vi "Feeding.vi"(8 "error In":errorcluster) -> (0 "error out":errorcluster)   [LabVIEW 2017]
uses:
  Controls/LOADING_DISPLAY.ctl
  <vilib>/Utility/error.llb/DialogType.ctl
  Controls/Feed_Cyc_Data.ctl
  Controls/QUEUE_STATES.ctl
  Controls/Feed_St.ctl
  <vilib>/Utility/file.llb/Read Delimited Spreadsheet (string).vi
  <vilib>/Instr/_visa.llb/VISA Configure Serial Port (Instr).vi
panel:
  out "ALL DOOR CLOSED":bool
  out "all rows":string[][](array[string])
  out "element":u16
  out "Boolean array":bool[](array[boolean])
  out "output cluster 2":cluster{"RECIPE INDEX":i32, "COMBI BIN":i32}
  in  "Close _Door":bool
  out "raw scan code":string
  in  "BYPASS SCN":bool
  in  "String":string
  out "Scanner Comm":bool
  out "Stop scanner":bool
  out "CYCLE STATUS":string
  out "CURRENT PLAN":T1
  out "SCAN CODE:":string
  out "Selected Plan structure":string[][](table)
  out "Plan Selected:":string
  out "USER:-":string
  in  "Stop":bool
  out "DATE/TIME":string
  out "Screen Name":string
  # "DOOR NUMBER"
  # "SCANNED CODE"
  # "FEEDER STATUS"
  # "DOOR NUMBER"
  # "SCANNED CODE"
  # "FEEDER STATUS"
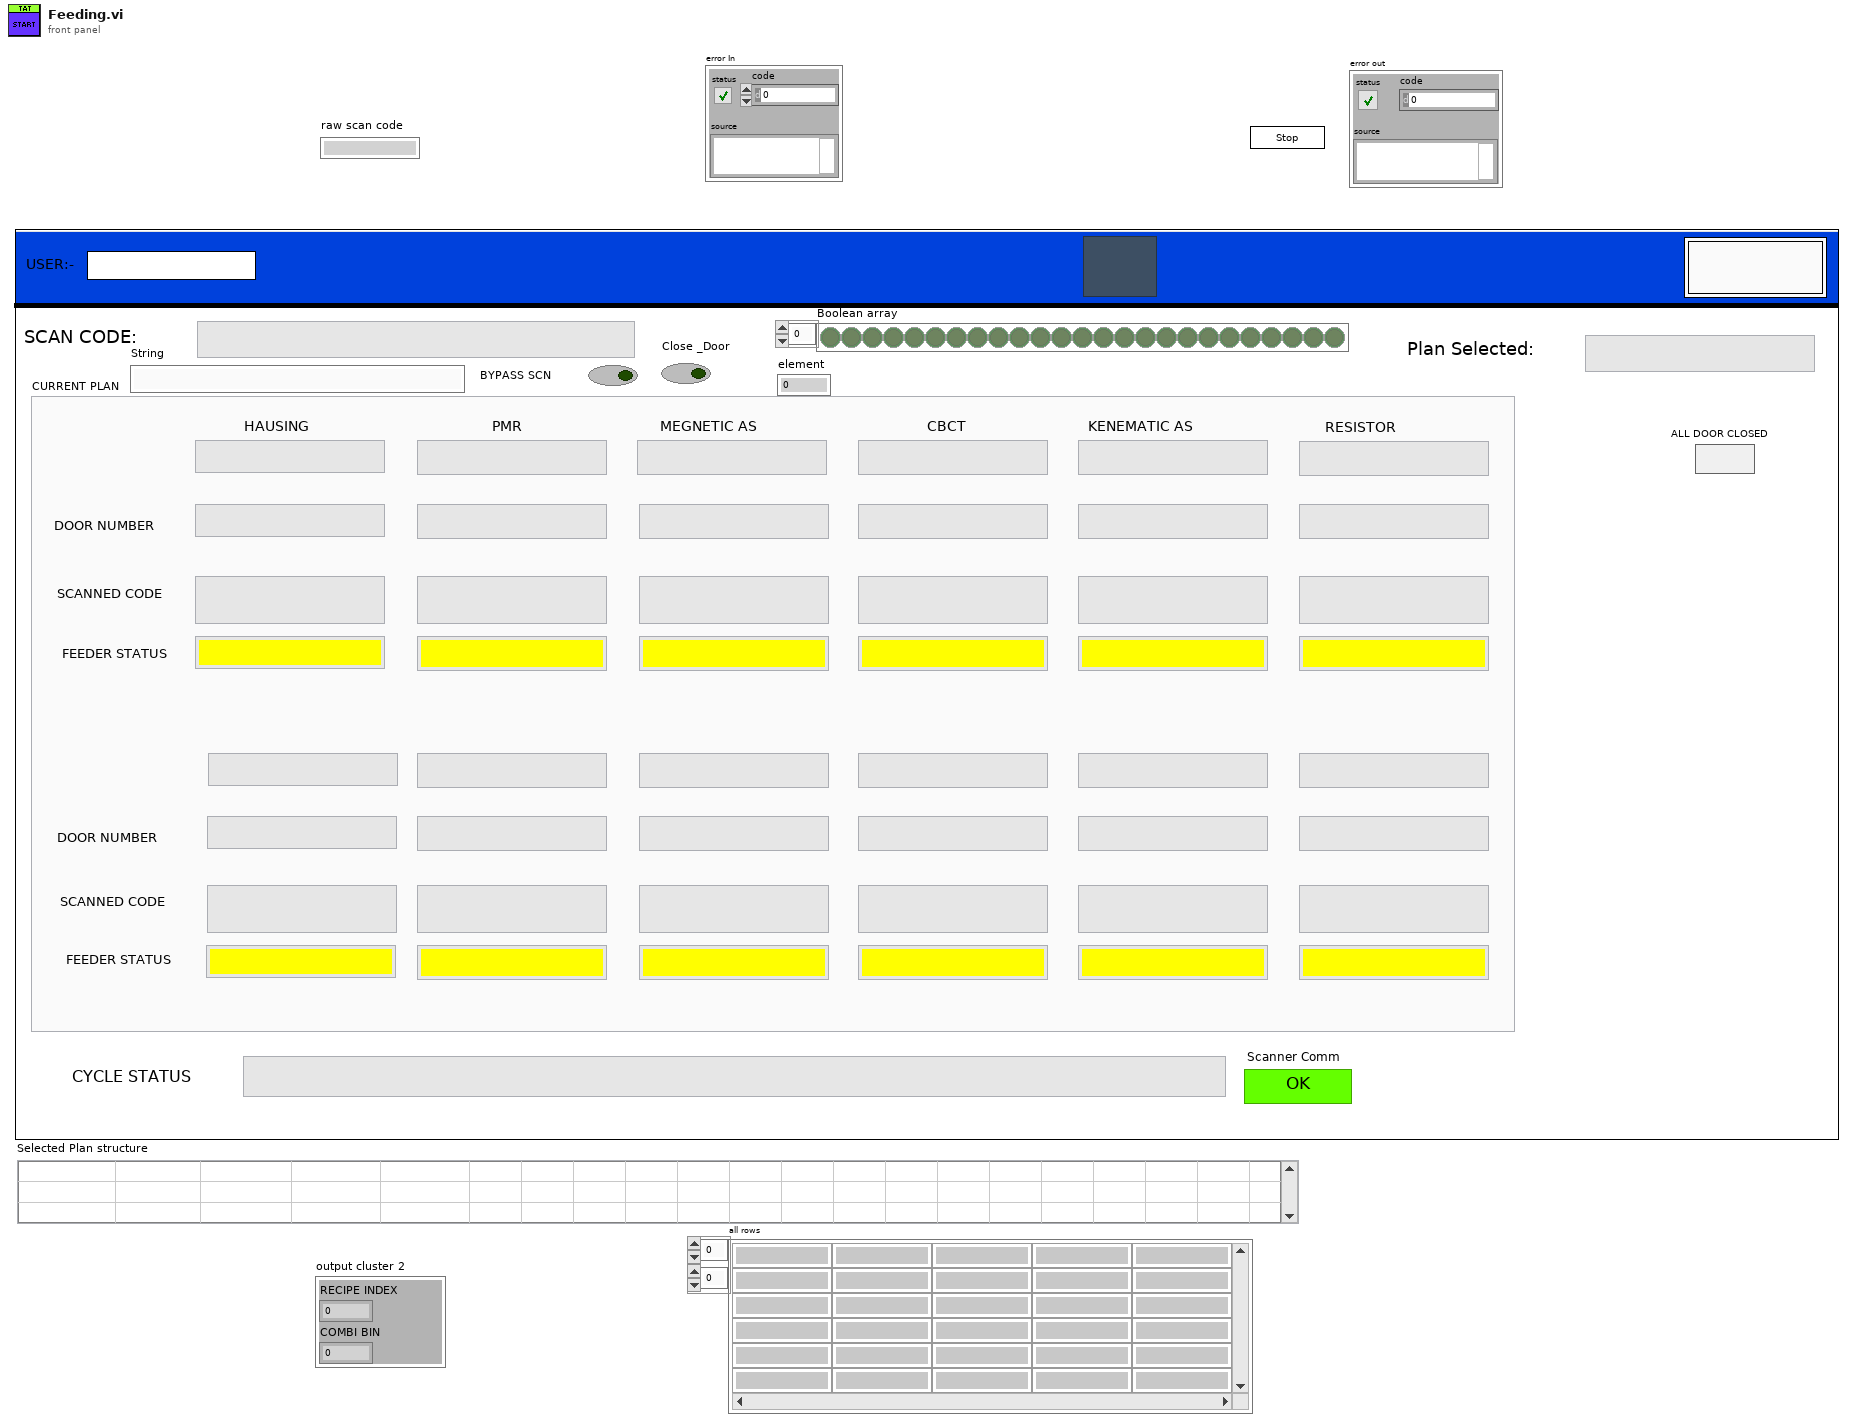
[diagram p1: front panel]
types:
  T1 = typedef "LOADING_DISPLAY.ctl" = cluster{"HAUSING":string, "PMR":string, "MEGNETIC AS":string, "CBCT":string, "KENEMATIC AS":string, "RESISTOR":string, "HAUSING DOOR":string, "PMR DOOR":string, "MAGNETIC AS DOOR":string, "CBCT DOOR":string, "KINEMATIC AS DOOR":string, "RESISTOR DOOR":string, "HAUSING SCAN QR":string, "PMR SCAN QR":string, "MAGNETIC SCAN QR":string, "CBCT SCAN QR":string, "KINEMATIC SCAN QR":string, "RESISTOR SCAN QR":string, "HAUSING FEED STATUS":string, "PMR FEED STATUS":string, "MAGNETIC AS FEEED STATUS":string, "CBCT FEED STATUS":string, "KINEMATIC AS FEED STATUS":string, "RESISTOR 1 FEED STATUS":string, "HAUSING 2":string, "PMR 2":string, "MEGNETIC AS 2":string, "CBCT 2":string, "KENEMATIC AS 2":string, "RESISTOR 2":string, "HAUSING DOOR 4":string, "PMR DOOR 4":string, "MAGNETIC AS DOOR 4":string, "CBCT DOOR 4":string, "KINEMATIC AS DOOR 4":string, "RESISTOR 1 DOOR 4":string, "HAUSING 2 SCAN QR":string, "PMR 2 SCAN QR":string, "MAGNETIC 2 SCAN QR":string, "CBCT 2 SCAN QR":string, "KINEMATIC 2 SCAN QR":string, "RESISTOR 2 SCAN QR":string, "HAUSING FEED STATUS 2":string, "PMR FEED STATUS 2":string, "MAGNETIC AS FEEED STATUS 2":string, "CBCT FEED STATUS 2":string, "KINEMATIC AS FEED STATUS 2":string, "RESISTOR 1 FEED STATUS 2":string}
  T2 = typedef "Feed_Cyc_Data.ctl" = cluster{"Cycle_Plan":path, "Plan_Data":string[][], "Scanned_Data":string[], "Scanned Chld Part":cluster{"Selected Door No":string, "child part code":string, "chld prt Row":i32, "Chld Prt Index":i32, "Scanned Data":string}, "feed Status Indi":refnum<vi>[], "Recipe Selected":cluster{"SELTED RECP & COMBI BIN":cluster{i32, i32}, "SELECTED RECIPE":string}, "CYCLE STATUS":string}
  T3 = typedef "DialogType.ctl" = u16
  T4 = enum32{"invalid app kind", "Development System", "Run Time System", "Student Edition", "Embedded LabVIEW", "Evaluation", "Custom"}
  T5 = typedef "QUEUE_STATES.ctl" = enum16{"CREATE Q", "EN Q", "DE Q", "CLOSE Q"}
  T6 = cluster{"Printer IP":string, "PLC IP Address":string, "Scanner Com":refnum<visa-resource-name>}
  T7 = typedef "Feed_St.ctl" = enum16{"Int 2", "Cluster_update", "Read_Plan", "QR_Scanned", "Int", "SaveReport ", "Error_Handler", "Wait", "Close_Door", "Stop"}
  T8 = cluster{"Selected Door No":string, "child part code":string, "chld prt Row":i32, "Chld Prt Index":i32, "Scanned Data":string}
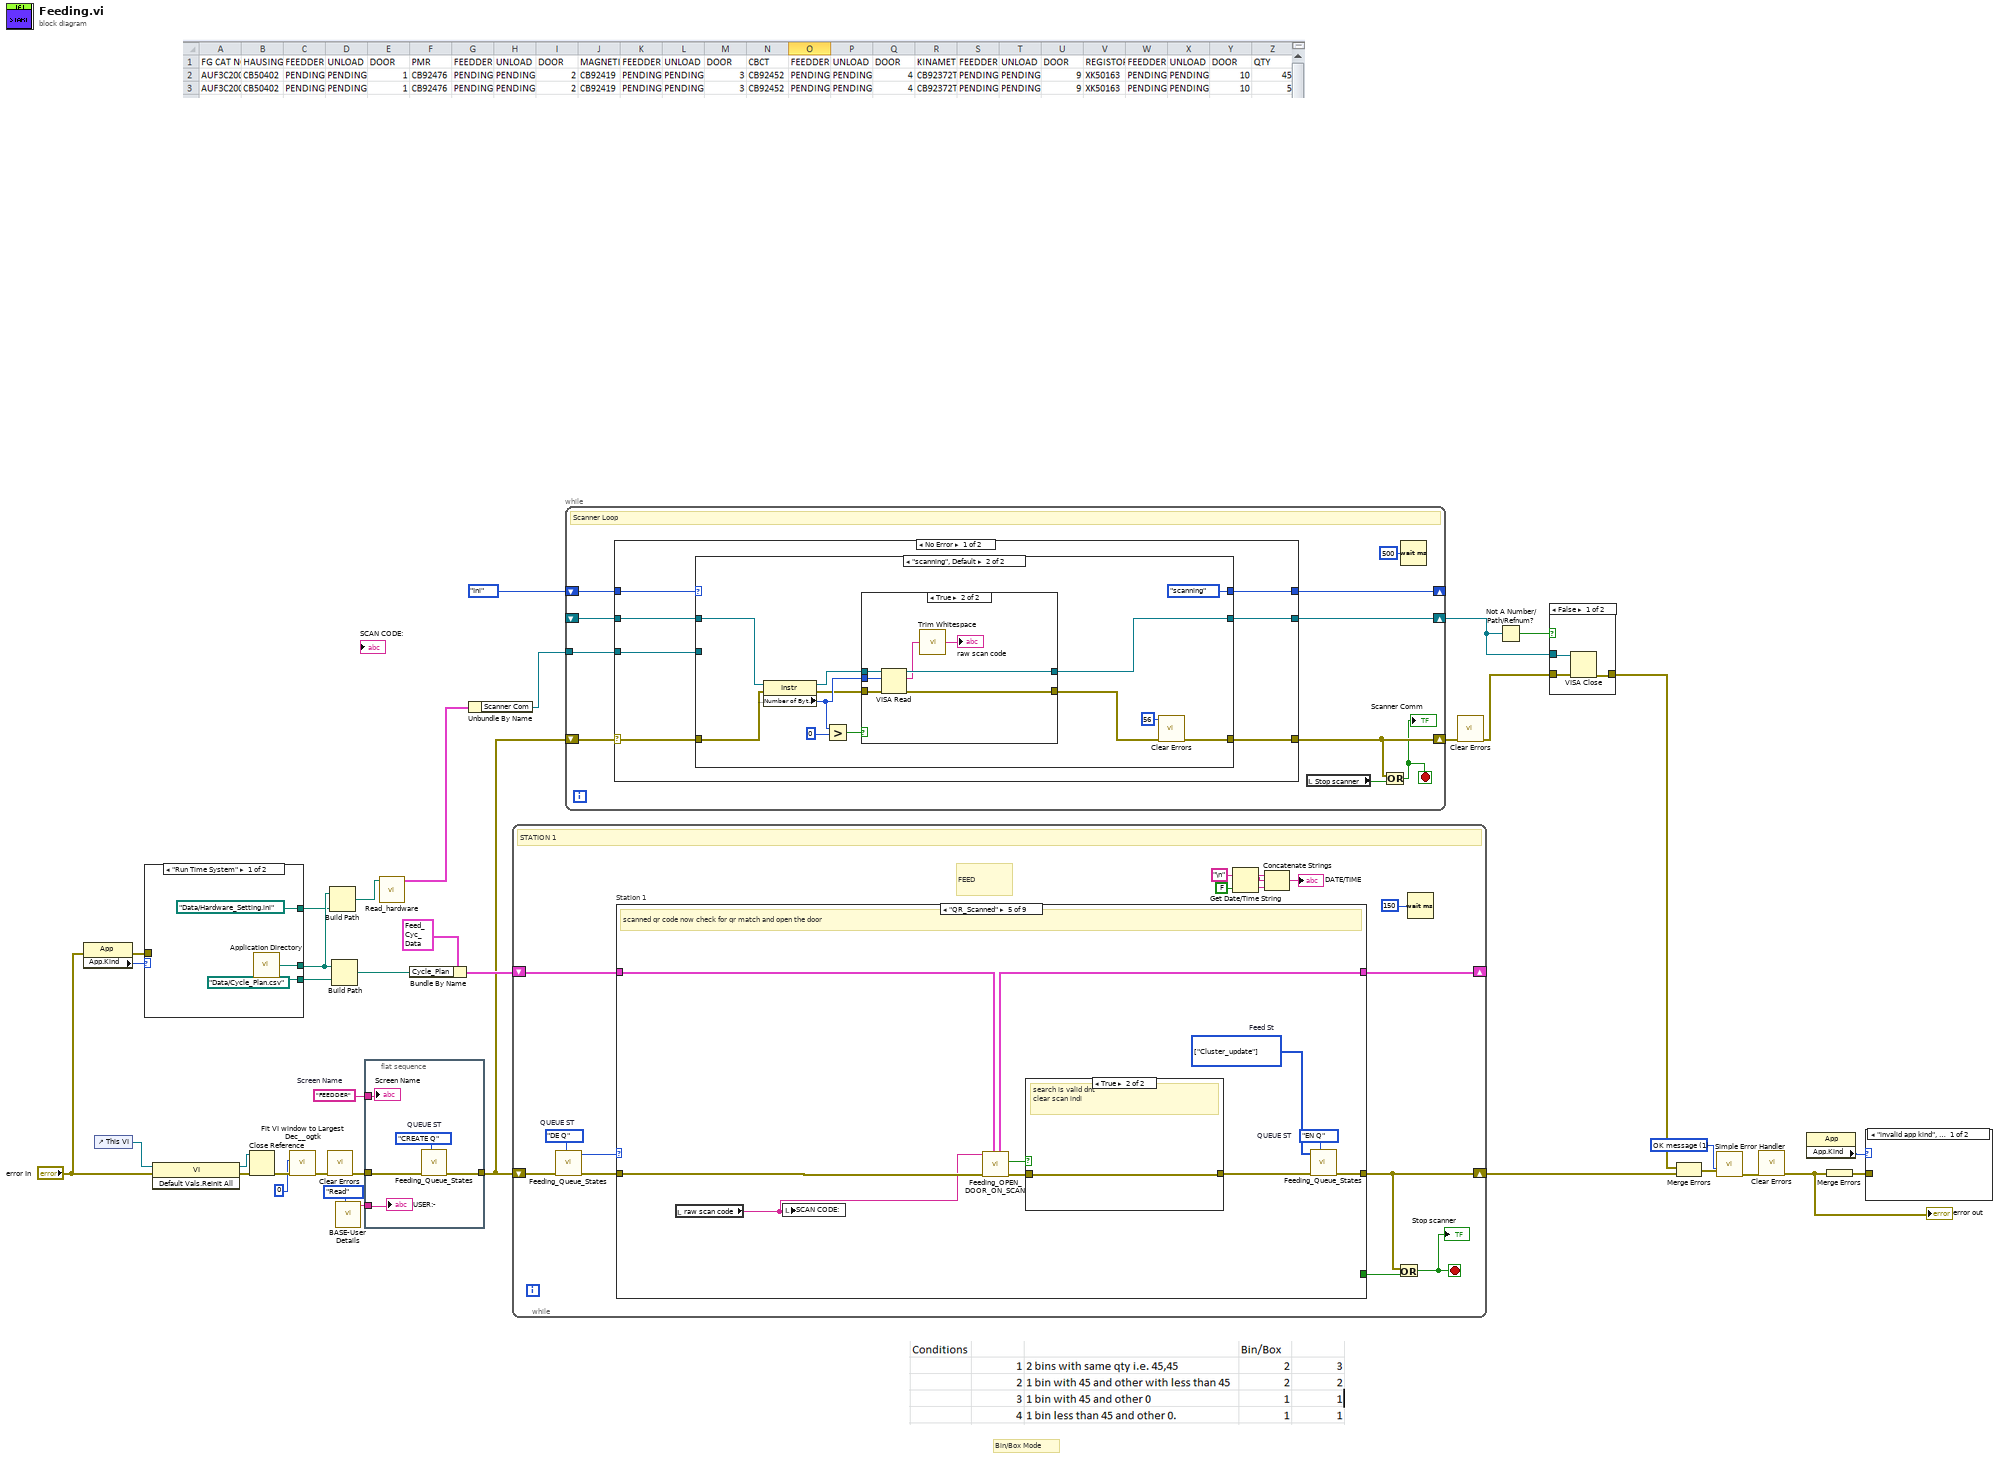
[diagram p0: block diagram]
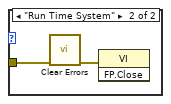
[diagram p2: hidden frame]
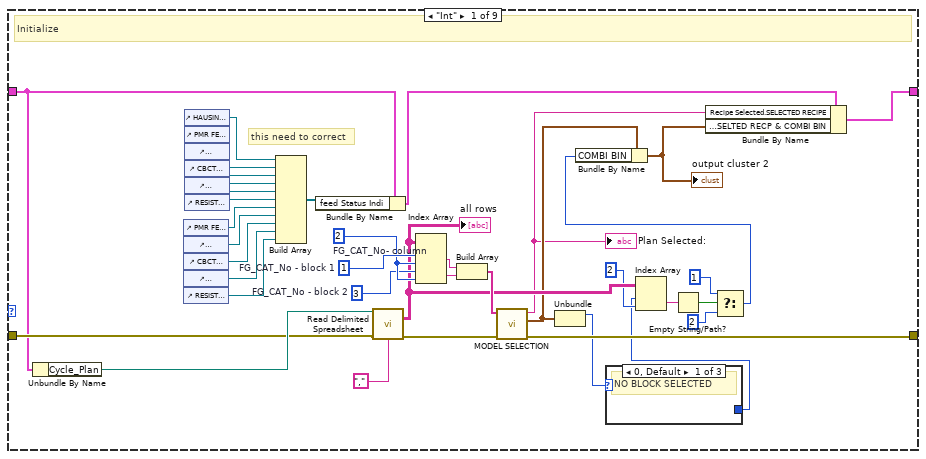
[diagram p3: hidden frame]
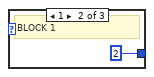
[diagram p4: hidden frame]
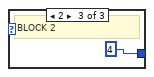
[diagram p5: hidden frame]
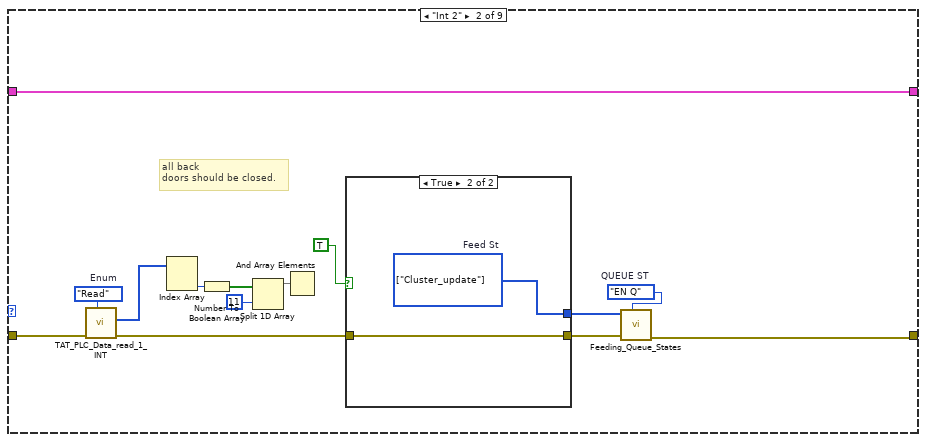
[diagram p6: hidden frame]
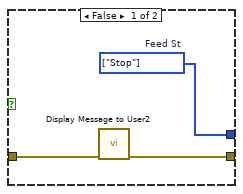
[diagram p7: hidden frame]
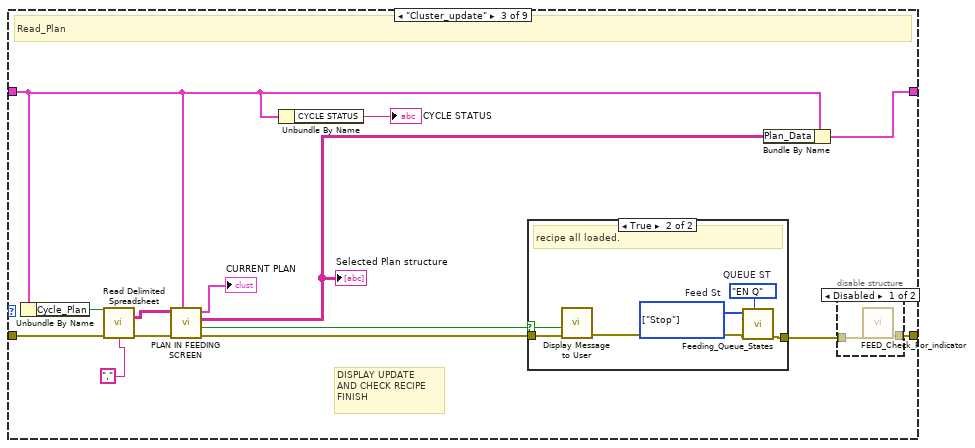
[diagram p8: hidden frame]
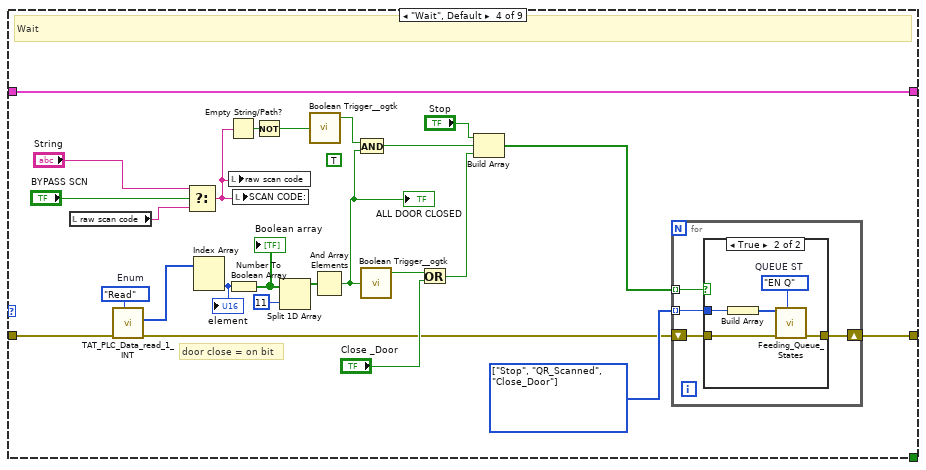
[diagram p11: hidden frame]
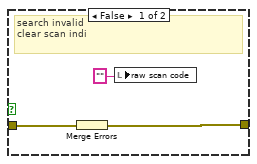
[diagram p13: hidden frame]
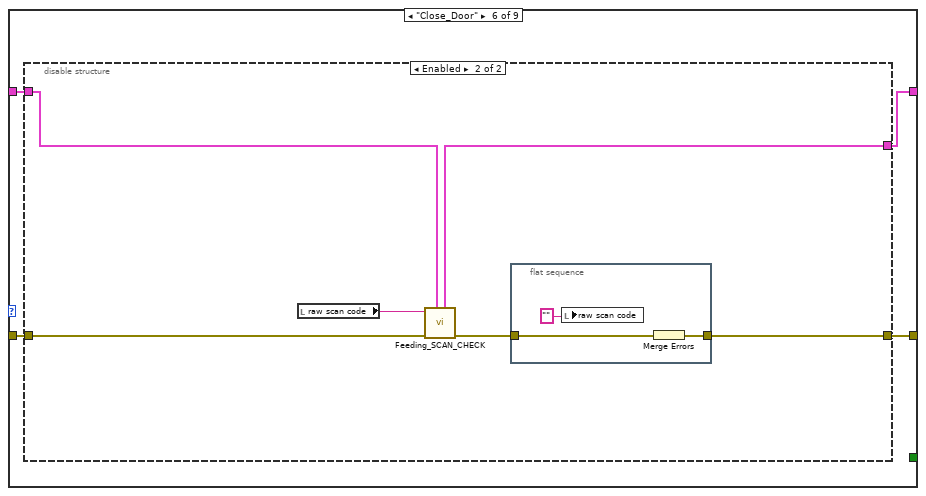
[diagram p14: hidden frame]
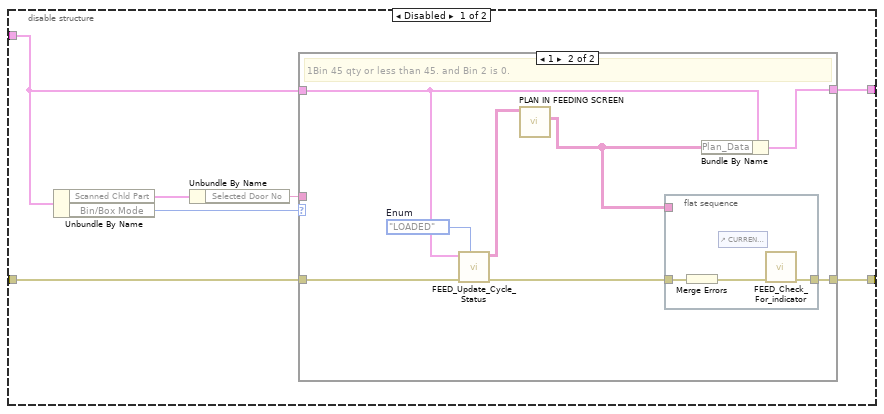
[diagram p15: hidden frame]
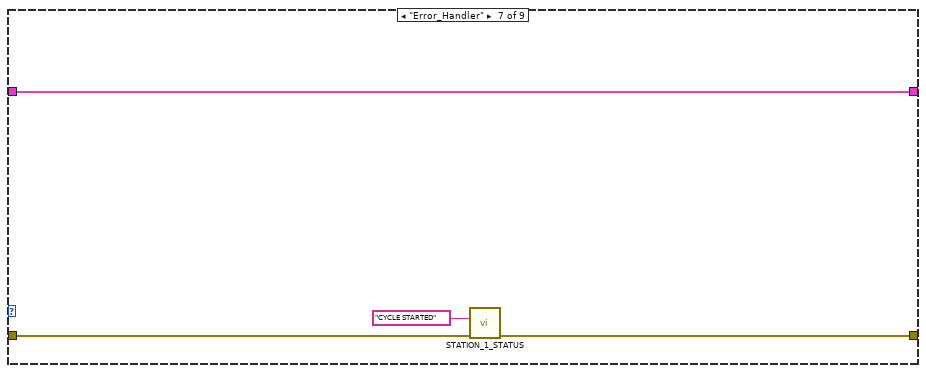
[diagram p17: hidden frame]
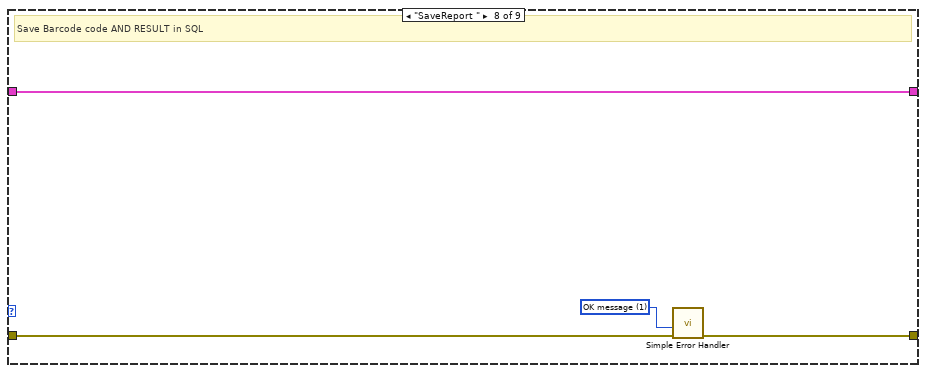
[diagram p18: hidden frame]
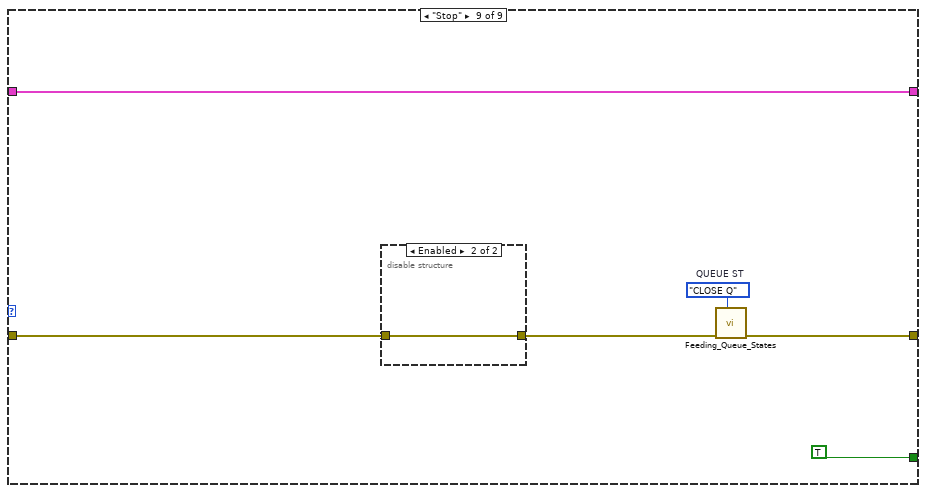
[diagram p19: hidden frame]
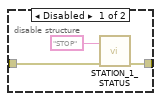
[diagram p20: hidden frame]
diagram:
  w17 = "FEEDDER"  # Screen Name
  w29 = T3 1 items=["no dialog", "OK message", "continue or stop message", "OK message + warnings", "continue/stop + warnings"] ("type of dialog (OK msg:1)")
  # "Bin/Box Mode"
  n1 = property class="App"(error in="error In") -> (error out=w25:errorcluster, "App.Kind"=w27:T4)  [unwired: 1 in, 1 out]
  n2 = control-ref of="This VI"() -> (w36:refnum<vi>)
  n3 = case shown="\"Run Time System\"" w27 {
    tunnel: [path "Data/Cycle_Plan.csv" ("path") path "../Data/Cycle_Plan.csv" ("path")] -> w26
    tunnel: [w37 w41] -> w6
    tunnel: w25 -> [_ _]
    tunnel: [path "Data/Hardware_Setting.ini" ("path") path "../Data/Hardware_Setting.ini" ("path")] -> w5
    frame "Run Time System" {
      n4 = call <vilib>:"Application Directory.vi"() -> ("Application Directory"=w37:path)
    }
    frame Default {
      n5 = Current VI's Path() -> (path=w42:path)
      n6 = Strip Path(path=w42) -> (stripped path=w41:path)  [unwired: 1 out]
    }
  }
  n7 = invoke class="VI" method="Default Vals.Reinit All"(reference=w36, error in="error In") -> (reference out=w34:refnum<vi>, error out=w35:errorcluster)  [unwired: 1 in, 1 out]
  n8 = Close Reference(reference=w34, error in (no error)=w35) -> (error out=w33:errorcluster)
  n9 = call <userlib>:"Fit VI window to Largest Dec__ogtk.vi"("error in (no error)"=w33, "border spacing (2 px)"=0) -> ("error out"=w23:errorcluster)  [unwired: 4 in, 1 out]
  n10 = call <vilib>:"Clear Errors.vi"("error in (no error)"=w23) -> ("error out"=w10:errorcluster)  [unwired: 5 in, 1 out]
  n11 = Build Path(base path=w6, name or relative path=w5) -> (appended path=w4:path)
  n12 = Build Path(base path=w6, name or relative path=w26) -> (appended path=w19:path)
  n13 = call "BASE-User Details.vi"("Enum"=enum16{"Read", "Write"}."Read") -> ("User Name Out"=w30:string)  [unwired: 9 in, 1 out]
  n14 = flat-sequence {
    tunnel: [w45] -> w11
    tunnel: w10 -> [w46]
    tunnel: w30 -> [w48]
    tunnel: w17 -> [w47]
    frame #0 {
      w44 = QUEUE_STATES."CREATE Q"  # QUEUE ST
      n15 = call "Feeding_Queue_States.vi"("QUEUE ST"=w44, "error in"=w46) -> ("error OUT"=w45:errorcluster)  [unwired: 8 in, 1 out]
      "USER:-" <- w48
      "Screen Name" <- w47
    }
  }
  n16 = call "Read_hardware.vi"("configuration file path"=w4) -> ("data"=w8:T6)  [unwired: 10 in]
  n17 = Bundle By Name(cluster=T2 {"Cycle_Plan"=path "", "Plan_Data"=[], "Scanned_Data"=[], "Scanned Chld Part"={"Selected Door No"="", "child part code"="", "chld prt Row"=0, "Chld Prt Index"=0, "Scanned Data"=""}, "feed Status Indi"=[], "Recipe Selected"={"SELTED RECP & COMBI BIN"={0, 0}, "SELECTED RECIPE"=""}, "CYCLE STATUS"=""}, "Cycle_Plan"=w19) -> (w18:T2)
  n18 = Unbundle By Name(w8) -> ("Scanner Com"=w7:refnum<visa-resource-name>)
  n19 = while {
    shift-right: [w55] -> _
    shift-left: w18 -> [w56]
    shift-right: [w53] -> w9
    shift-left: w11 -> [w52]
    stop <- w54 stop-if-true
    w50 = QUEUE_STATES."DE Q"  # QUEUE ST
    # "FEED"
    # "STATION 1"
    n20 = call "Feeding_Queue_States.vi"("QUEUE ST"=w50, "error in"=w52) -> ("error OUT"=w51:errorcluster, "Feed ST"=w49:T7)  [unwired: 8 in]
    n21 = case "Station 1" shown="\"QR_Scanned\"" w49 {
      tunnel: [_ _ _ _ _ _ _ _ TRUE] -> w57
      tunnel: [w67 w106 w130 w168 w183 w198 w230 w235 w237] -> w53
      tunnel: w51 -> [w86 w110 w135 w157 w191 w199 w231 w234 w241]
      tunnel: w56 -> [w77 w117 w124 w171 w188 w197 w229 w233 w240]
      tunnel: [w78 w117 w129 w171 w187 w196 w229 w233 w240] -> w55
      frame "Int" {
        w82 = 3  # FG_CAT_No - block 2
        w84 = 1  # FG_CAT_No - block 1
        w83 = 2  # FG_CAT_No- column
        # "this need to correct"
        # "Initialize"
        n22 = Unbundle By Name(w77) -> ("Cycle_Plan"=w89:path)
        n23 = control-ref of="PMR FEED STATUS 2"() -> (w97:refnum<vi>)
        n24 = control-ref of="MAGNETIC AS FEEED STATUS 2"() -> (w98:refnum<vi>)
        n25 = control-ref of="CBCT FEED STATUS 2"() -> (w99:refnum<vi>)
        n26 = control-ref of="KINEMATIC AS FEED STATUS 2"() -> (w100:refnum<vi>)
        n27 = control-ref of="RESISTOR 1 FEED STATUS 2"() -> (w101:refnum<vi>)
        n28 = control-ref of="HAUSING FEED STATUS"() -> (w91:refnum<vi>)
        n29 = control-ref of="PMR FEED STATUS"() -> (w92:refnum<vi>)
        n30 = control-ref of="MAGNETIC AS FEEED STATUS"() -> (w93:refnum<vi>)
        n31 = control-ref of="CBCT FEED STATUS"() -> (w94:refnum<vi>)
        n32 = control-ref of="KINEMATIC AS FEED STATUS"() -> (w95:refnum<vi>)
        n33 = control-ref of="RESISTOR 1 FEED STATUS"() -> (w96:refnum<vi>)
        n34 = Build Array(w91, w92, w93, w94, w95, w96, w97, w98, w99, w100, w101) -> (w90:refnum<vi>[])
        n35 = Bundle By Name(cluster=w77, "feed Status Indi"=w90) -> (w79:T2)
        n36 = call-poly <vilib>:"Read Delimited Spreadsheet.vi"("file path (dialog if empty)"=w89, "error in (no error)"=w86, "delimiter (\\t)"=",") -> ("all rows"=w76:string[][], "error out"=w85:errorcluster)  [unwired: 7 in, 4 out]
        "all rows" <- w76
        n37 = Index Array(array=w76, index (row) #1=w84, index (col) #1=w83, index (row) #2=w82, index (col) #2=w83) -> (element #1=w81:string, element #2=w80:string)
        n38 = Build Array(w81, w80) -> (w88:string[])
        n39 = call "MODEL SELECTION.vi"("error in (no error)"=w85, "Plan List"=w88) -> ("error out 2"=w67:errorcluster, "SELECTED RECIPE\nand COMBI OF BIN- INDEX"=w70:cluster{"RECIPE INDEX":i32, "COMBI BIN":i32}, "Plan Selected"=w68:string)  [unwired: 7 in]
        "Plan Selected:" <- w68
        n40 = Unbundle(w70) -> ("RECIPE INDEX"=w66:i32)  [unwired: 1 out]
        n41 = case shown="0, Default" w66 {
          tunnel: [_ 2 4] -> w64
          frame 0, Default {
            # "NO BLOCK SELECTED"
          }
          frame 1 {
            # "BLOCK 1"
          }
          frame 2 {
            # "BLOCK 2"
          }
        }
        n42 = Index Array(array=w76, index (row)=w64, index (col)=2) -> (element=w74:string)
        n43 = Empty String/Path?(string/path=w74) -> (empty?=w73:bool)
        n44 = Select(t=1, s=w73, f=2) -> (s? t:f=w65:i32)
        n45 = Bundle By Name(cluster=w70, "COMBI BIN"=w65) -> (w69:cluster{"RECIPE INDEX":i32, "COMBI BIN":i32})
        "output cluster 2" <- w69
        n46 = Bundle By Name(cluster=w79, "Recipe Selected.SELECTED RECIPE"=w68, "Recipe Selected.SELTED RECP & COMBI BIN"=w69) -> (w78:T2)
      }
      frame "Int 2" {
        w108 = QUEUE_STATES."EN Q"  # QUEUE ST
        w116 = enum16{"Read", "Write"}."Read"  # Enum
        # "all back\ndoors should be closed."
        n47 = call "TAT_PLC_Data_read_1_INT.vi"("Enum"=w116, "error in (no error)"=w110) -> ("error out"=w109:errorcluster, "Array 2"=w115:u16[])  [unwired: 8 in]
        n48 = Index Array(array=w115) -> (element #2=w114:u16)  [unwired: 2 in, 1 out]
        n49 = Number To Boolean Array(number=w114) -> (Boolean array=w113:bool[])
        n50 = Split 1D Array(array=w113, index=11) -> (first subarray=w111:bool[])  [unwired: 1 out]
        n51 = And Array Elements(Boolean array=w111) -> ()  [unwired: 1 out]
        n52 = case shown="True" TRUE {
          tunnel: w109 -> [w119 w121]
          tunnel: [w118 w121] -> w105
          tunnel: [w120 w122] -> w107
          frame False {
            w120 = T7[] [enum."Stop"] items=["Int 2", "Cluster_update", "Read_Plan", "QR_Scanned", "Int", "SaveReport ", "Error_Handler", "Wait", "Close_Door", "Stop"]  # Feed St
            n53 = call "Display Message to User2"("error in (no error)"=w119) -> ("error out"=w118:errorcluster)  [unwired: 9 in, 1 out]
          }
          frame True {
            w122 = T7[] [enum."Cluster_update"] items=["Int 2", "Cluster_update", "Read_Plan", "QR_Scanned", "Int", "SaveReport ", "Error_Handler", "Wait", "Close_Door", "Stop"]  # Feed St
          }
        }
        n54 = call "Feeding_Queue_States.vi"("QUEUE ST"=w108, "error in"=w105, "Feed St"=w107) -> ("error OUT"=w106:errorcluster)  [unwired: 7 in, 1 out]
      }
      frame "Cluster_update" {
        # "DISPLAY UPDATE\nAND CHECK RECIPE\nFINISH"
        # "Read_Plan"
        n55 = Unbundle By Name(w124) -> ("Cycle_Plan"=w134:path)
        n56 = call-poly <vilib>:"Read Delimited Spreadsheet.vi"("file path (dialog if empty)"=w134, "error in (no error)"=w135, "delimiter (\\t)"=",") -> ("all rows"=w132:string[][], "error out"=w127:errorcluster)  [unwired: 7 in, 4 out]
        n57 = call "PLAN IN FEEDING SCREEN.vi"("LOOP DATA IN"=w124, "error IN"=w127, "PLAN In"=w132) -> ("error out"=w128:errorcluster, "NO EMPTY CMPLT?"=w125:bool, "PLAN Out"=w133:string[][], "CURRENT PLAN"=→"CURRENT PLAN":T1)  [unwired: 4 in]
        "Selected Plan structure" <- w133
        n58 = Unbundle By Name(w124) -> ("CYCLE STATUS"=→"CYCLE STATUS":string)
        n59 = case shown="True" w125 {
          selector: w125 -> [_ w141]
          tunnel: w128 -> [w140 w143]
          tunnel: [w140 w145] -> w131
          frame False {
          }
          frame True {
            w144 = T7[] [enum."Stop"] items=["Int 2", "Cluster_update", "Read_Plan", "QR_Scanned", "Int", "SaveReport ", "Error_Handler", "Wait", "Close_Door", "Stop"]  # Feed St
            w146 = QUEUE_STATES."EN Q"  # QUEUE ST
            # "recipe all loaded."
            n60 = call "Display Message to User"("error in (no error)"=w143, "Enable"=w141) -> ("error out"=w142:errorcluster)  [unwired: 8 in, 1 out]
            n61 = call "Feeding_Queue_States.vi"("QUEUE ST"=w146, "error in"=w142, "Feed St"=w144) -> ("error OUT"=w145:errorcluster)  [unwired: 7 in, 1 out]
          }
        }
        n62 = Bundle By Name(cluster=w124, "Plan_Data"=w133) -> (w129:T2)
        n63 = disable-structure shown="Disabled" {
          disable-tunnel: w131 -> [w138 w139]
          disable-tunnel: [w137 w139] -> w130
          frame Disabled {
            n64 = call "FEED_Check_For_indicator.vi"("error in (no error)"=w138) -> ("error out"=w137:errorcluster)  [unwired: 10 in]
          }
          frame Enabled {
          }
        }
      }
      frame "Wait", Default {
        (unwired) TRUE
        w155 = enum16{"Read", "Write"}."Read"  # Enum
        w164 = T7[] [enum."Stop", enum."QR_Scanned", enum."Close_Door"] items=["Int 2", "Cluster_update", "Read_Plan", "QR_Scanned", "Int", "SaveReport ", "Error_Handler", "Wait", "Close_Door", "Stop"] ("Array")
        # "door close = on bit"
        # "Wait"
        n65 = local read "raw scan code"() -> (w163:string)
        n66 = call "TAT_PLC_Data_read_1_INT.vi"("Enum"=w155, "error in (no error)"=w157) -> ("error out"=w156:errorcluster, "Array 2"=w154:u16[])  [unwired: 8 in]
        n67 = Select(t="String", s="BYPASS SCN", f=w163) -> (s? t:f=w160:string)
        n68 = Index Array(array=w154) -> (element #2=w151:u16)  [unwired: 2 in, 1 out]
        "element" <- w151
        n69 = Empty String/Path?(string/path=w160) -> (empty?=w167:bool)
        n70 = local write "raw scan code"(w160) -> ()
        n71 = Number To Boolean Array(number=w151) -> (Boolean array=w150:bool[])
        "Boolean array" <- w150
        n72 = local write "SCAN CODE:"(w160) -> ()
        n73 = Not(x=w167) -> (.not. x?=w159:bool)
        n74 = Split 1D Array(array=w150, index=11) -> (first subarray=w148:bool[])  [unwired: 1 out]
        n75 = call <userlib>:"Boolean Trigger__ogtk.vi"("Boolean Input"=w159) -> ("Rising Edge"=w158:bool)  [unwired: 1 in, 1 out]
        n76 = And Array Elements(Boolean array=w148) -> (logical AND=w147:bool)
        "ALL DOOR CLOSED" <- w147
        n77 = And(x=w158, y=w147) -> (x .and. y?=w153:bool)
        n78 = call <userlib>:"Boolean Trigger__ogtk.vi"("Boolean Input"=w147) -> ("Rising Edge"=w152:bool)  [unwired: 1 in, 1 out]
        n79 = Or(x=w152, y="Close _Door") -> (x .or. y?=w161:bool)
        n80 = Build Array("Stop", w153, w161) -> (w165:bool[])
        n81 = for {
          shift-right: [w174] -> w168
          shift-left: w156 -> [w175]
          tunnel: w165 -> [w173] mode=indexing
          tunnel: w164 -> [w172] mode=indexing
          n82 = case shown="True" w173 {
            tunnel: w175 -> [w176 w180]
            tunnel: [w176 w179] -> w174
            tunnel: w172 -> [_ w178]
            frame False {
            }
            frame True {
              w181 = QUEUE_STATES."EN Q"  # QUEUE ST
              n83 = Build Array(w178) -> (w177:T7[])
              n84 = call "Feeding_Queue_States.vi"("QUEUE ST"=w181, "error in"=w180, "Feed St"=w177) -> ("error OUT"=w179:errorcluster)  [unwired: 7 in, 1 out]
            }
          }
        }
      }
      frame "QR_Scanned" {
        w184 = T7[] [enum."Cluster_update"] items=["Int 2", "Cluster_update", "Read_Plan", "QR_Scanned", "Int", "SaveReport ", "Error_Handler", "Wait", "Close_Door", "Stop"]  # Feed St
        w185 = QUEUE_STATES."EN Q"  # QUEUE ST
        # "scanned qr code now check for qr match and open the door"
        n85 = local read "raw scan code"() -> (w189:string)
        n86 = local write "SCAN CODE:"(w189) -> ()
        n87 = call "Feeding_OPEN_DOOR_ON_SCAN.vi"("CYCLE DATA IN"=w188, "error in (no error)"=w191, "raw scan code"=w189) -> ("error out"=w190:errorcluster, "search valid ?"=w186:bool, "CYCLE DATA OUT"=w187:T2)  [unwired: 6 in]
        n88 = case shown="True" w186 {
          tunnel: w190 -> [w194 w195]
          tunnel: [w193 w195] -> w182
          frame False {
            # "search invalid\nclear scan indi"
            n89 = Merge Errors(w194) -> (w193:errorcluster)
            n90 = local write "raw scan code"("") -> ()
          }
          frame True {
            # "search is valid dnt\nclear scan indi"
          }
        }
        n91 = call "Feeding_Queue_States.vi"("QUEUE ST"=w185, "error in"=w182, "Feed St"=w184) -> ("error OUT"=w183:errorcluster)  [unwired: 7 in, 1 out]
      }
      frame "Close_Door" {
        n92 = disable-structure shown="Enabled" {
          disable-tunnel: w199 -> [w206 w225]
          disable-tunnel: [w205 w220] -> w198
          disable-tunnel: w197 -> [w202 w223]
          disable-tunnel: [w201 w222] -> w196
          frame Disabled {
            n93 = Unbundle By Name(w202) -> ("Scanned Chld Part"=w203:T8, "Bin/Box Mode"=w200:i32)
            n94 = Unbundle By Name(w203) -> ("Selected Door No"=w204:string)
            n95 = case shown="1" w200 {
              tunnel: w206 -> [w207 w215]
              tunnel: [w207 w210] -> w205
              tunnel: w204 -> [_ _]
              tunnel: w202 -> [w208 w212]
              tunnel: [w208 w216] -> w201
              frame 0, Default {
              }
              frame 1 {
                w213 = enum16{"FEED", "LOADED"}."LOADED"  # Enum
                # "1Bin 45 qty or less than 45. and Bin 2 is 0."
                n96 = call "FEED_Update_Cycle_Status.vi"("Enum"=w213, "error in (no error)"=w215, 11:w212) -> ("error out"=w214:errorcluster, "output array"=w211:string[][])  [unwired: 6 in, 1 out]
                n97 = call "PLAN IN FEEDING SCREEN.vi"("PLAN In"=w211) -> ("PLAN Out"=w209:string[][])  [unwired: 6 in, 3 out]
                n98 = flat-sequence {
                  tunnel: w214 -> [w219]
                  tunnel: [w217] -> w210
                  tunnel: w209 -> [_]
                  frame #0 {
                    n99 = Merge Errors(w219) -> (w218:errorcluster)
                    n100 = control-ref of="CURRENT PLAN"() -> ()  [unwired: 1 out]
                    n101 = call "FEED_Check_For_indicator.vi"("error in (no error)"=w218) -> ("error out"=w217:errorcluster)  [unwired: 10 in]
                  }
                }
                n102 = Bundle By Name(cluster=w212, "Plan_Data"=w209) -> (w216:T2)
              }
            }
          }
          frame Enabled {
            n103 = local read "raw scan code"() -> (w221:string)
            n104 = call "Feeding_SCAN_CHECK.vi"("CYCLE DATA IN"=w223, "error in (no error)"=w225, "raw scan code"=w221) -> ("error out"=w224:errorcluster, "CYCLE DATA OUT"=w222:T2)  [unwired: 7 in]
            n105 = flat-sequence {
              tunnel: w224 -> [w228]
              tunnel: [w226] -> w220
              frame #0 {
                n106 = local write "raw scan code"("") -> ()
                n107 = Merge Errors(w228) -> (w226:errorcluster)
              }
            }
          }
        }
      }
      frame "Error_Handler" {
        n108 = call "STATION_1_STATUS.vi"("error in (no error)"=w231, "STATUS"="CYCLE STARTED" ("Cycle Status")) -> ("error out"=w230:errorcluster)  [unwired: 9 in]
      }
      frame "SaveReport " {
        w236 = T3 1 items=["no dialog", "OK message", "continue or stop message", "OK message + warnings", "continue/stop + warnings"] ("type of dialog (OK msg:1)")
        # "Save Barcode code AND RESULT in SQL"
        n109 = call <vilib>:"Simple Error Handler.vi"("type of dialog (OK msg:1)"=w236, "error in (no error)"=w234) -> ("error out"=w235:errorcluster)  [unwired: 3 in, 4 out]
      }
      frame "Stop" {
        w239 = QUEUE_STATES."CLOSE Q"  # QUEUE ST
        n110 = disable-structure shown="Enabled" {
          disable-tunnel: w241 -> [w244 w246]
          disable-tunnel: [w243 w246] -> w238
          frame Disabled {
            n111 = call "STATION_1_STATUS.vi"("error in (no error)"=w244, "STATUS"="STOP" ("Cycle Status")) -> ("error out"=w243:errorcluster)  [unwired: 9 in]
          }
          frame Enabled {
          }
        }
        n112 = call "Feeding_Queue_States.vi"("QUEUE ST"=w239, "error in"=w238) -> ("error OUT"=w237:errorcluster)  [unwired: 8 in, 1 out]
      }
    }
    n113 = Get Date/Time String(want seconds? (F)=FALSE) -> (date string=w61:string, time string=w60:string)  [unwired: 2 in]
    n114 = Concatenate Strings(w61, "\n", w60) -> (→"DATE/TIME":string)
    n115 = Or(x=w53, y=w57) -> (x .or. y?=w54:bool)
    "Stop scanner" <- w54
    n116 = Wait (ms)(milliseconds to wait=u32 150) -> ()  [unwired: 1 out]
  }
  n117 = while {
    shift-right: [w255] -> w15
    shift-left: w11 -> [w256]
    shift-right: [w253] -> _
    shift-left: enum16{"Ini", "scanning", "Close"}."Ini" -> [w254]
    tunnel: w7 -> [w252]
    shift-right: [w251] -> w12
    shift-left: _ -> [w250]
    stop <- w249 stop-if-true
    # "Scanner Loop"
    n118 = case shown="No Error" w256 {
      selector: w256 -> [w263 w293]
      tunnel: [w262 w292] -> w255
      tunnel: w254 -> [w261 _]
      tunnel: [w260 enum16{"Ini", "scanning", "Close"}."scanning"] -> w253
      tunnel: w252 -> [w259 _]
      tunnel: [w258 w290] -> w251
      tunnel: w250 -> [w257 w290]
      frame No Error {
        n119 = case shown="\"scanning\", Default" w261 {
          tunnel: w263 -> [w267 w271]
          tunnel: [w266 w279] -> w262
          tunnel: [enum16{"Ini", "scanning", "Close"}."scanning" enum16{"Ini", "scanning", "Close"}."scanning"] -> w260
          tunnel: w259 -> [w265 _]
          tunnel: [w264 w269] -> w258
          tunnel: w257 -> [_ w272]
          frame "Ini" {
            n120 = call-poly "VISA Configure Serial Port"("VISA resource name"=w265, "error in (no error)"=w267) -> ("VISA resource name out"=w264:refnum<visa-resource-name>, "error out"=w266:errorcluster)  [unwired: 12 in]
          }
          frame "scanning", Default {
            n121 = property class="Instr"(reference=w272, error in=w271) -> (reference out=w274:refnum<visa-resource-name>, error out=w275:errorcluster, "Serial Settings:Number of Bytes at Serial Port"=w276:u32)
            n122 = Greater?(x=w276, y=u32 0) -> (0:w277:bool)
            n123 = case shown="True" w277 {
              tunnel: w274 -> [w282 w289]
              tunnel: w275 -> [w281 w288]
              tunnel: w276 -> [_ w287]
              tunnel: [w282 w286] -> w269
              tunnel: [w281 w284] -> w270
              frame False {
              }
              frame True {
                n124 = VISA Read(VISA resource name=w289, byte count=w287, error in (no error)=w288) -> (VISA resource name out=w286:refnum<visa-resource-name>, read buffer=w285:string, error out=w284:errorcluster)  [unwired: 1 out]
                n125 = call <vilib>:"Trim Whitespace.vi"("string"=w285) -> ("trimmed string"=→"raw scan code":string)  [unwired: 1 in]
              }
            }
            n126 = call <vilib>:"Clear Errors.vi"("error in (no error)"=w270, "specific error code to clear (0: all)"=56) -> ("error out"=w279:errorcluster)  [unwired: 4 in, 1 out]
          }
        }
      }
      frame Error {
        n127 = Unbundle By Name(w293) -> ("code"=w294:i32)
        n128 = case shown="1" w294 {
          tunnel: w293 -> [w298 w300]
          tunnel: [w296 w299] -> w292
          frame 0, Default {
            w295 = T3 2 items=["no dialog", "OK message", "continue or stop message", "OK message + warnings", "continue/stop + warnings"] ("type of dialog (OK msg:1)")
            n129 = call <vilib>:"Simple Error Handler.vi"("type of dialog (OK msg:1)"=w295, "error in (no error)"=w298) -> ("error out"=w297:errorcluster)  [unwired: 3 in, 4 out]
            n130 = call <vilib>:"Clear Errors.vi"("error in (no error)"=w297) -> ("error out"=w296:errorcluster)  [unwired: 5 in, 1 out]
          }
          frame 1 {
            w301 = "THIS ERROR OCCURED AS SCREEN 1 IS NOT CONNECTED OR OFF"  # source
            # "Monitor not present/Off/disconnected"
            n131 = Bundle By Name(cluster=w300, "source"=w301) -> (w299:errorcluster)
          }
        }
      }
    }
    n132 = local read "Stop scanner"() -> (w247:bool)
    n133 = Or(x=w255, y=w247) -> (x .or. y?=w249:bool)
    "Scanner Comm" <- w249
    n134 = Wait (ms)(milliseconds to wait=u32 500) -> ()  [unwired: 1 out]
  }
  n135 = call <vilib>:"Clear Errors.vi"("error in (no error)"=w15) -> ("error out"=w13:errorcluster)  [unwired: 5 in, 1 out]
  n136 = Not A Number/Path/Refnum?(number/path/refnum=w12) -> (NaN/Path/Refnum?=w14:bool)
  n137 = case shown="False" w14 {
    tunnel: w13 -> [w304 w305]
    tunnel: w12 -> [w302 _]
    tunnel: [w303 w305] -> w3
    frame False {
      n138 = VISA Close(VISA resource name=w302, error in (no error)=w304) -> (error out=w303:errorcluster)
    }
    frame True {
    }
  }
  n139 = Merge Errors(w3, w9) -> (w32:errorcluster)
  n140 = call <vilib>:"Simple Error Handler.vi"("type of dialog (OK msg:1)"=w29, "error in (no error)"=w32) -> ("error out"=w2:errorcluster)  [unwired: 3 in, 4 out]
  n141 = call <vilib>:"Clear Errors.vi"("error in (no error)"=w2) -> ("error out"=w1:errorcluster)  [unwired: 5 in, 1 out]
  "error out" <- w1
  n142 = property class="App"() -> ("App.Kind"=w28:T4)  [unwired: 2 in, 2 out]
  n143 = Merge Errors(w1) -> (w21:errorcluster)
  n144 = case shown="\"invalid app kind\", Default" w28 {
    tunnel: w21 -> [_ w307]
    frame "invalid app kind", Default {
    }
    frame "Run Time System" {
      n145 = call <vilib>:"Clear Errors.vi"("error in (no error)"=w307) -> ("error out"=w306:errorcluster)  [unwired: 5 in, 1 out]
      n146 = invoke class="VI" method="FP.Close"(error in=w306) -> ()  [unwired: 2 in, 3 out]
    }
  }
